vi "Stability Tracker.vi"(0 "Tolerance":dbl, 1 "AbsError":dbl, 2 "PI Running?":bool, 5 "ReqReads":i32, 7 "Parameter":i32, 9 "Setpoint":dbl format="%#_13g", 11 "StabilityCount In":i32) -> (8 "Stable?":bool, 15 "StabilityCount Out":i32)   [LabVIEW 2013]
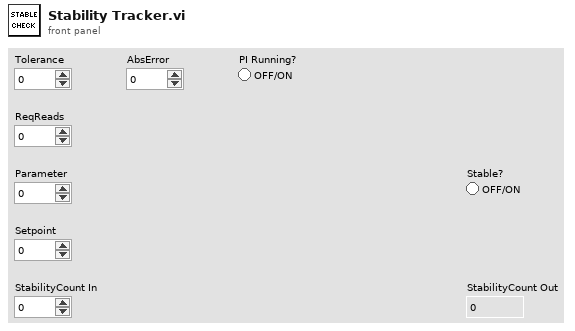
[diagram p1: front panel]
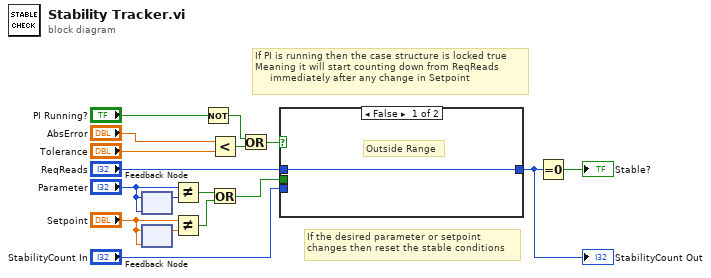
[diagram p0: block diagram]
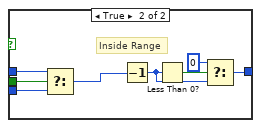
[diagram p2: hidden frame]
diagram:
  # "If PI is running then the case structure is locked true\nMeaning it will start counting down from ReqReads\n     immediately after any change in Setpoint"
  # "If the desired parameter or setpoint\nchanges then reset the stable conditions"
  n1 = feedback #1("Parameter") -> (w11:i32)
  n2 = feedback-in #1("Parameter") -> ()
  n3 = feedback #2("Setpoint") -> (w12:dbl)
  n4 = feedback-in #2("Setpoint") -> ()
  n5 = Not Equal?(x="Parameter", y=w11) -> (x != y?=w13:bool)
  n6 = Not Equal?(x="Setpoint", y=w12) -> (x != y?=w14:bool)
  n7 = Not(x="PI Running?") -> (.not. x?=w15:bool)
  n8 = Less?(x="AbsError", y="Tolerance") -> (x < y?=w16:bool)
  n9 = Or(x=w13, y=w14) -> (x .or. y?=w10:bool)
  n10 = Or(x=w15, y=w16) -> (x .or. y?=w17:bool)
  n11 = case shown="False" w17 {
    tunnel: [w18 w23] -> w6
    tunnel: "ReqReads" -> [w18 w21]
    tunnel: w10 -> [_ w22]
    tunnel: "StabilityCount In" -> [_ w19]
    frame False {
      # "Outside Range"
    }
    frame True {
      # "Inside Range"
      n12 = Select(t=w21, s=w22, f=w19) -> (s? t:f=w20:i32)
      n13 = Decrement(x=w20) -> (x-1=w25:i32)
      n14 = Less Than 0?(x=w25) -> (x < 0?=w24:bool)
      n15 = Select(t=0, s=w24, f=w25) -> (s? t:f=w23:i32)
    }
  }
  "StabilityCount Out" <- w6
  n16 = Equal To 0?(x=w6) -> (x = 0?=→"Stable?":bool)
